vi "Clear Memory.vi"(8 "error in (no error)":errorcluster, 10 "Memory (0: All)":u16(ring) items=["All", "Memory 1", "Memory 2", "Memory 3", "Memory 4"], 11 "VISA resource name":refnum<visa-resource-name>) -> (0 "error out":errorcluster, 3 "VISA resource name out":refnum<visa-resource-name>)   [LabVIEW 2013, in "LeCroy Wave Series.lvlib"]
doc: "This clear specified memory or all memories together."
uses:
  LeCroy Wave Series.lvlib
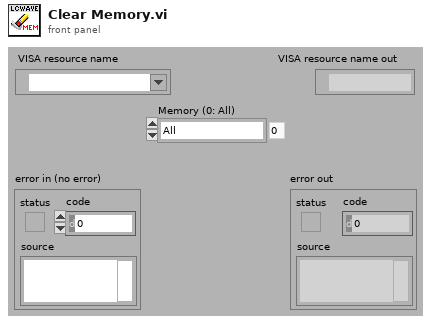
[diagram p1: front panel]
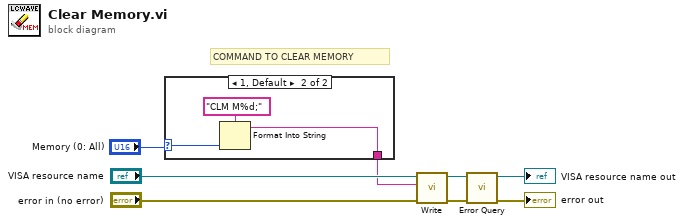
[diagram p0: block diagram]
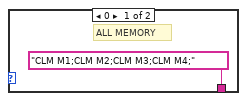
[diagram p2: hidden frame]
diagram:
  # "COMMAND TO CLEAR MEMORY"
  n1 = case shown="1, Default" "Memory (0: All)" {
    selector: "Memory (0: All)" -> [_ w11]
    tunnel: ["CLM M1;CLM M2;CLM M3;CLM M4;" w10] -> w1
    frame 0 {
      # "ALL MEMORY"
    }
    frame 1, Default {
      n2 = Format Into String(format string="CLM M%d;", w11) -> (resulting string=w10:string)  [unwired: 2 in, 1 out]
    }
  }
  n3 = call "Write.vi"("error in (no error)"="error in (no error)", "Write Buffer"=w1, "VISA resource name"="VISA resource name") -> ("error out"=w3:errorcluster, "VISA resource name out"=w4:refnum<visa-resource-name>)  [unwired: 6 in, 1 out]
  n4 = call "Error Query.vi"("error in (no error)"=w3, "VISA resource name"=w4) -> ("error out"=→"error out":errorcluster, "VISA resource name out"=→"VISA resource name out":refnum<visa-resource-name>)  [unwired: 6 in, 2 out]
